vi "set_spiral_params.vi"(8 "error in (no error)":errorcluster, 9 "dump factor":dbl, 10 "Spiral":bool, 11 "TrajectoryTS090820Circular2D in":refnum<class "TrajectoryTS090820Circular2D.lvclass">) -> (0 "error out":errorcluster, 3 "TrajectoryTS090820Circular2D out":refnum<class "TrajectoryTS090820Circular2D.lvclass">)   [LabVIEW 2010, in "TrajectoryTS090820Circular2D.lvclass"]
uses:
  TrajectoryTS090820Circular2D.lvclass
  TrajectoryTS090820Circular2D.lvclass/TrajectoryTS090820Circular2D.ctl
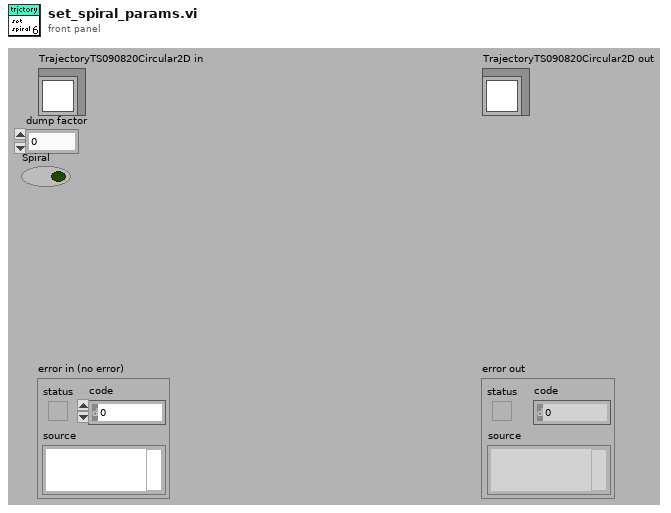
[diagram p1: front panel]
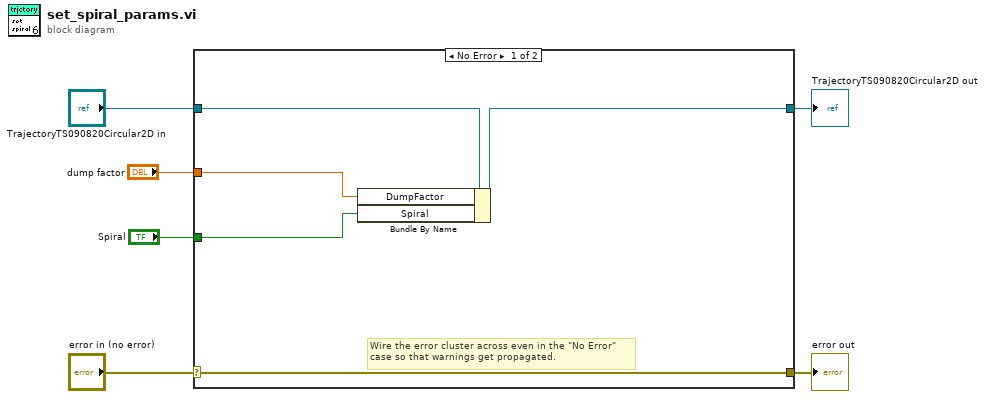
[diagram p0: block diagram]
diagram:
  n1 = case shown="No Error" "error in (no error)" {
    selector: "error in (no error)" -> [w11 w13]
    tunnel: [w11 w13] -> w5
    tunnel: [w9 w12] -> w3
    tunnel: "TrajectoryTS090820Circular2D in" -> [w10 w12]
    tunnel: "Spiral" -> [w8 _]
    tunnel: "dump factor" -> [w7 _]
    frame No Error {
      # "Wire the error cluster across even in the \"No Error\"\ncase so that warnings get propagated."
      n2 = Bundle By Name(cluster=w10, "DumpFactor"=w7, "Spiral"=w8) -> (w9:refnum<class "TrajectoryTS090820Circular2D.lvclass">)
    }
    frame Error {
    }
  }
  "error out" <- w5
  "TrajectoryTS090820Circular2D out" <- w3
